vi "practice-01_thirteen segment display.vi"() -> ()   [LabVIEW 2015]
panel:
  out "Boolean 13":bool
  out "Boolean 12":bool
  out "Boolean 11":bool
  out "Boolean 3":bool
  out "Boolean 10":bool
  in  "stop 2":bool
  out "Boolean 6":bool
  out "Boolean 5":bool
  out "Boolean 7":bool
  out "Boolean 4":bool
  out "Boolean 8":bool
  out "Boolean 2":bool
  out "Boolean 9":bool
  in  "interlock":bool
  in  "emg2":bool
  in  "stop":bool
  in  "net":bool
  out "lamp":bool
  in  "emg1\nemg1":bool
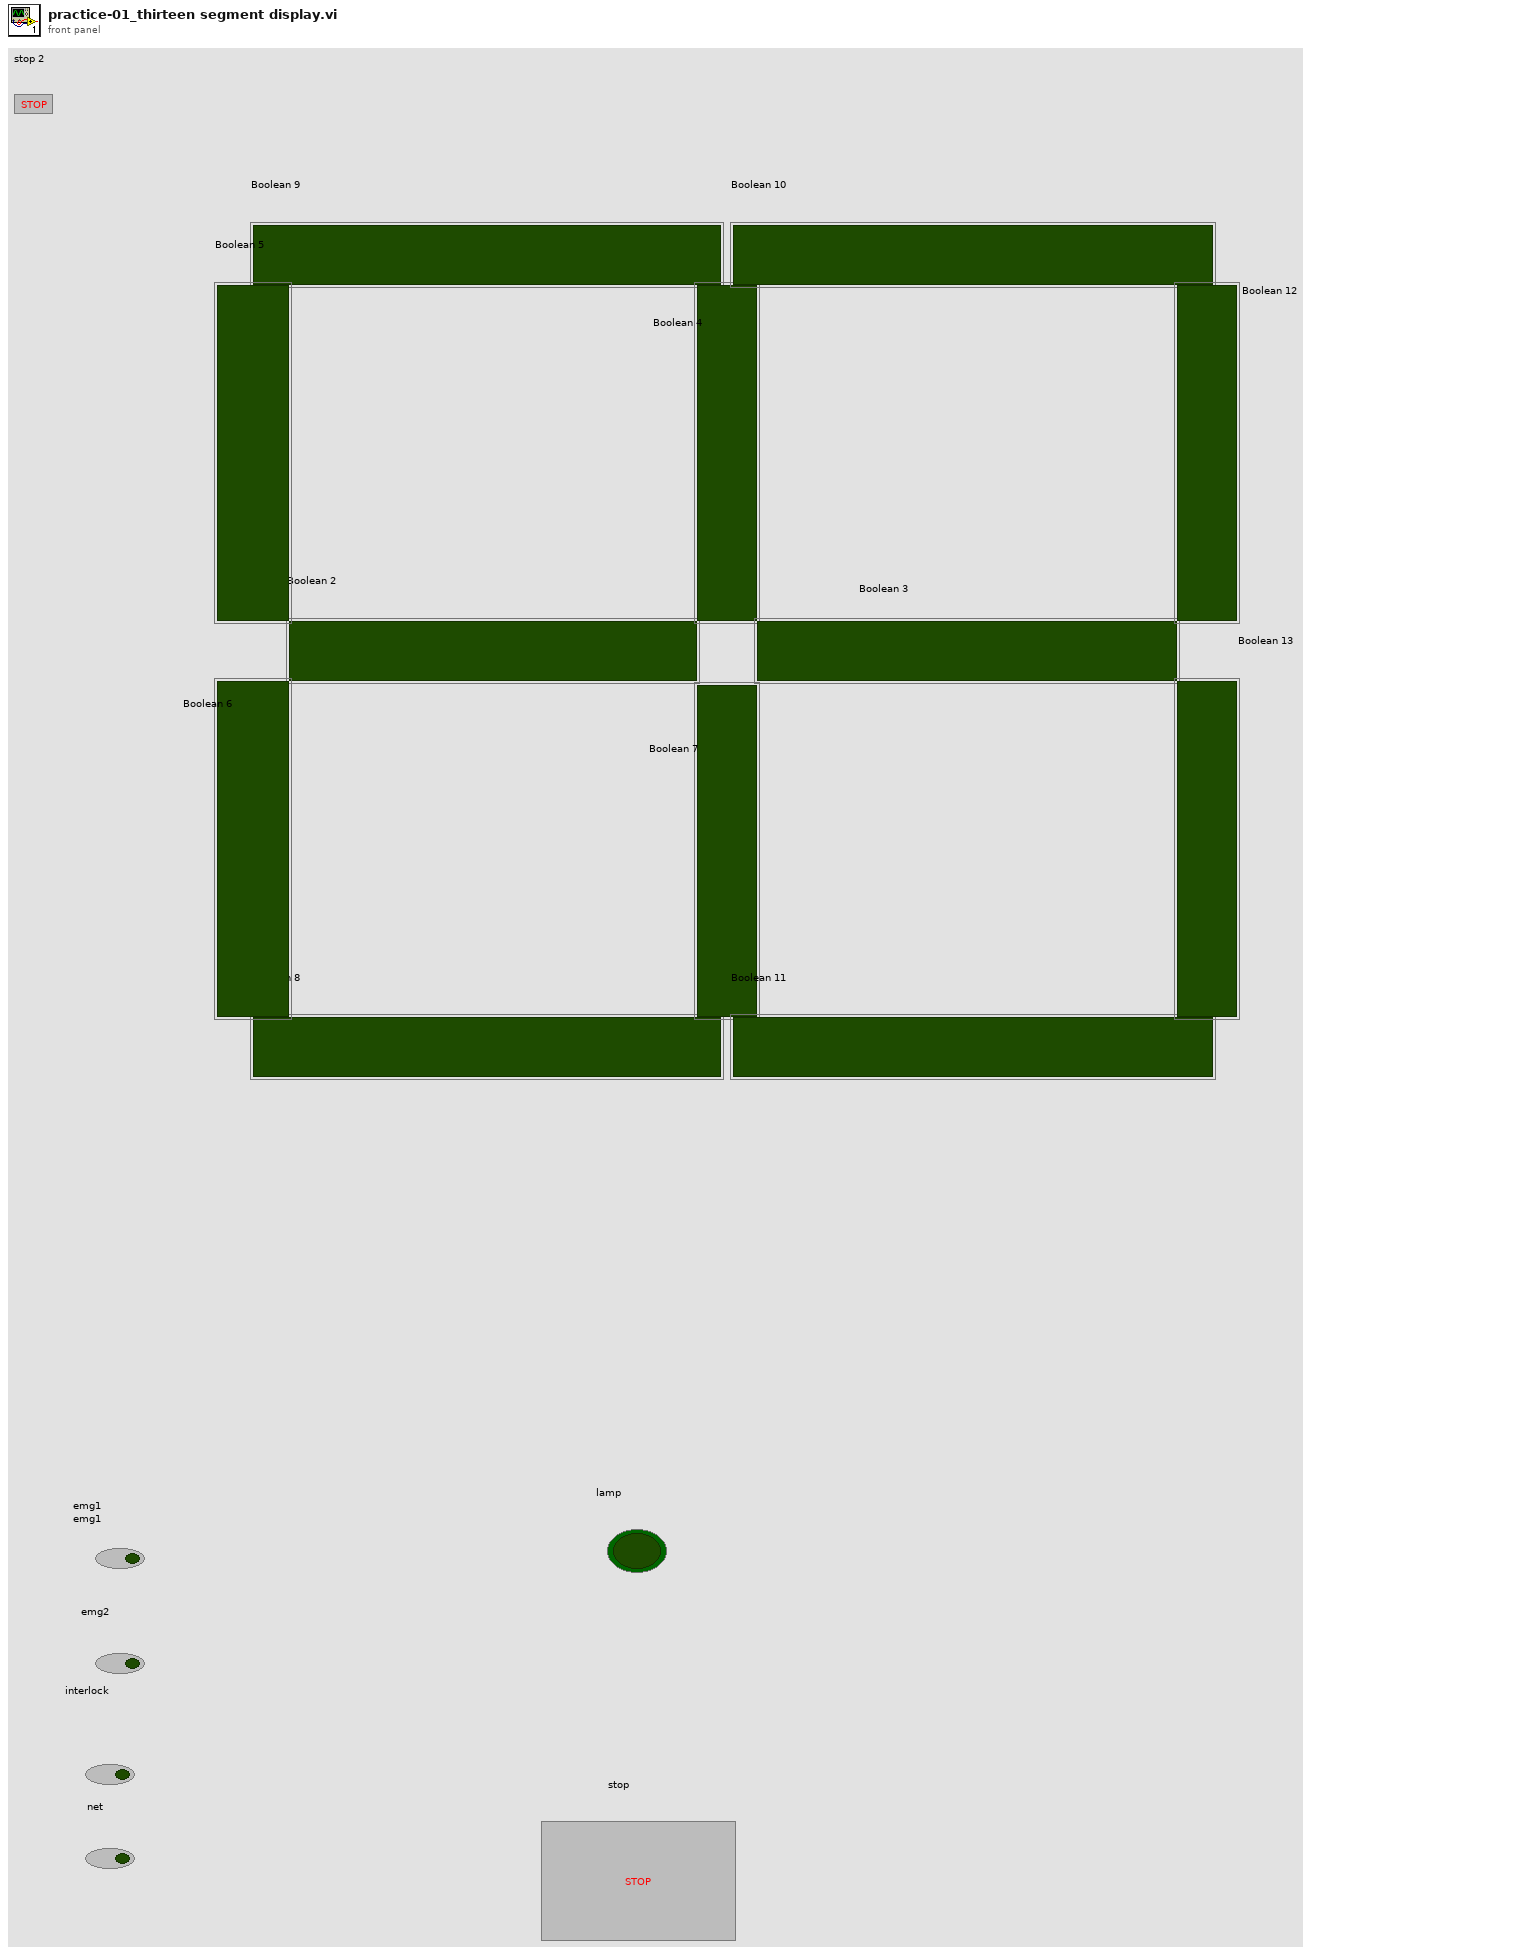
[diagram p1: front panel]
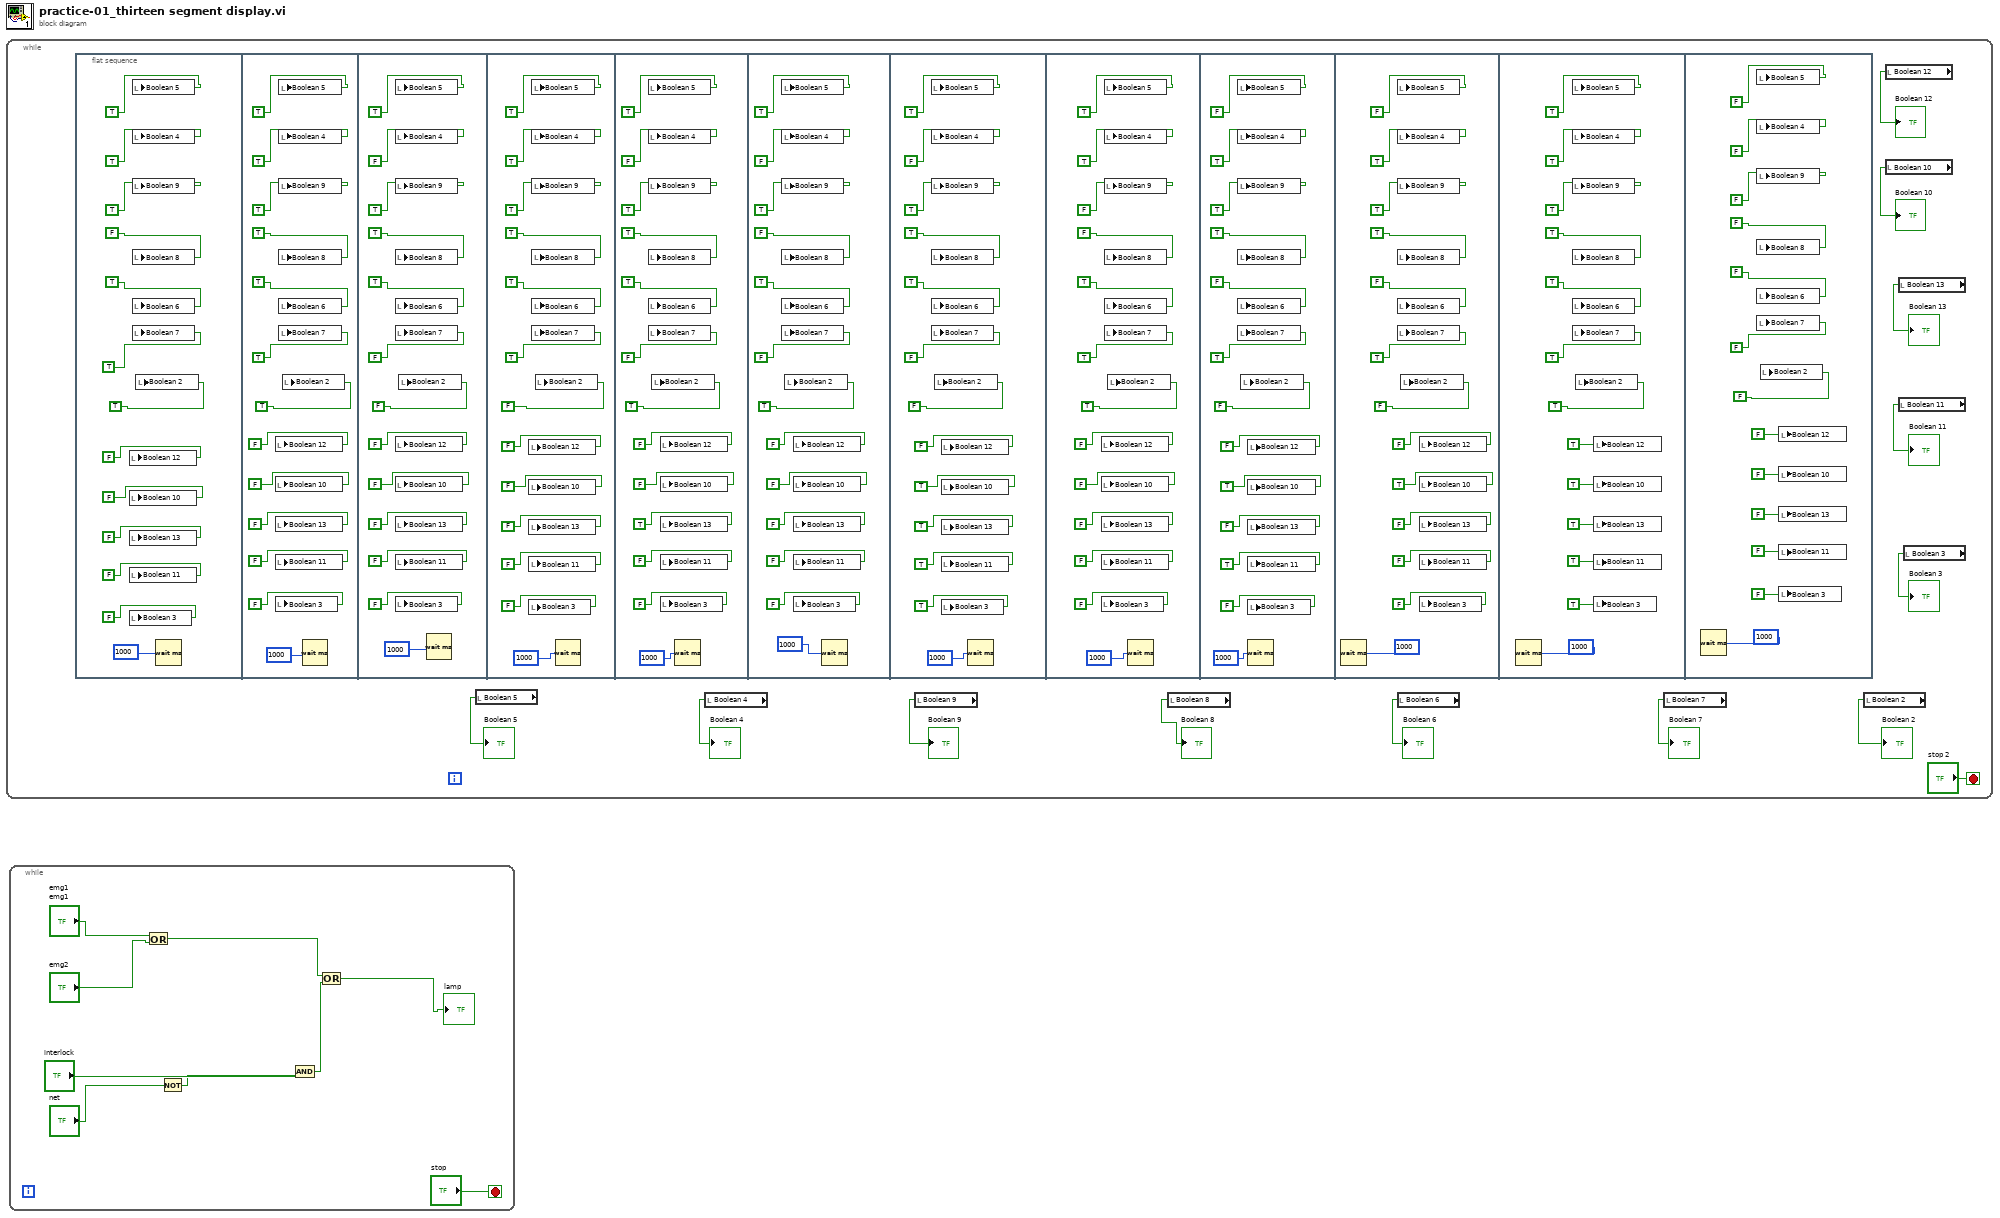
[diagram p0: block diagram]
diagram:
  n1 = while {
    stop <- "stop 2" stop-if-true
    n2 = flat-sequence {
      frame #0 {
        n3 = local write "Boolean 12"(FALSE ("Boolean 12")) -> ()
        n4 = local write "Boolean 10"(FALSE ("Boolean 10")) -> ()
        n5 = local write "Boolean 13"(FALSE ("Boolean 13")) -> ()
        n6 = local write "Boolean 11"(FALSE ("Boolean 11")) -> ()
        n7 = local write "Boolean 3"(FALSE ("Boolean 3")) -> ()
        n8 = local write "Boolean 5"(TRUE ("Boolean 5")) -> ()
        n9 = local write "Boolean 4"(TRUE ("Boolean 4")) -> ()
        n10 = local write "Boolean 9"(TRUE ("Boolean 9")) -> ()
        n11 = local write "Boolean 8"(FALSE ("Boolean 8")) -> ()
        n12 = local write "Boolean 6"(TRUE ("Boolean 5")) -> ()
        n13 = local write "Boolean 7"(TRUE ("Boolean 7")) -> ()
        n14 = local write "Boolean 2"(TRUE ("Boolean 2")) -> ()
        n15 = Wait (ms)(milliseconds to wait=u32 1000 ("millisecond timer value")) -> ()  [unwired: 1 out]
      }
      frame #1 {
        n16 = local write "Boolean 12"(FALSE ("Boolean 12")) -> ()
        n17 = local write "Boolean 10"(FALSE ("Boolean 10")) -> ()
        n18 = local write "Boolean 13"(FALSE ("Boolean 13")) -> ()
        n19 = local write "Boolean 11"(FALSE ("Boolean 11")) -> ()
        n20 = local write "Boolean 3"(FALSE ("Boolean 3")) -> ()
        n21 = local write "Boolean 5"(TRUE ("Boolean 5")) -> ()
        n22 = local write "Boolean 4"(TRUE ("Boolean 4")) -> ()
        n23 = local write "Boolean 9"(TRUE ("Boolean 9")) -> ()
        n24 = local write "Boolean 8"(TRUE ("Boolean 8")) -> ()
        n25 = local write "Boolean 6"(TRUE ("Boolean 5")) -> ()
        n26 = local write "Boolean 7"(TRUE ("Boolean 7")) -> ()
        n27 = local write "Boolean 2"(TRUE ("Boolean 2")) -> ()
        n28 = Wait (ms)(milliseconds to wait=u32 1000 ("millisecond timer value")) -> ()  [unwired: 1 out]
      }
      frame #2 {
        n29 = local write "Boolean 5"(TRUE ("Boolean 5")) -> ()
        n30 = local write "Boolean 4"(FALSE ("Boolean 4")) -> ()
        n31 = local write "Boolean 9"(TRUE ("Boolean 9")) -> ()
        n32 = local write "Boolean 8"(TRUE ("Boolean 8")) -> ()
        n33 = local write "Boolean 6"(TRUE ("Boolean 5")) -> ()
        n34 = local write "Boolean 7"(FALSE ("Boolean 7")) -> ()
        n35 = local write "Boolean 12"(FALSE ("Boolean 12")) -> ()
        n36 = local write "Boolean 10"(FALSE ("Boolean 10")) -> ()
        n37 = local write "Boolean 13"(FALSE ("Boolean 13")) -> ()
        n38 = local write "Boolean 11"(FALSE ("Boolean 11")) -> ()
        n39 = local write "Boolean 3"(FALSE ("Boolean 3")) -> ()
        n40 = local write "Boolean 2"(FALSE ("Boolean 2")) -> ()
        n41 = Wait (ms)(milliseconds to wait=u32 1000 ("millisecond timer value")) -> ()  [unwired: 1 out]
      }
      frame #3 {
        n42 = local write "Boolean 12"(FALSE ("Boolean 12")) -> ()
        n43 = local write "Boolean 10"(FALSE ("Boolean 10")) -> ()
        n44 = local write "Boolean 13"(FALSE ("Boolean 13")) -> ()
        n45 = local write "Boolean 11"(FALSE ("Boolean 11")) -> ()
        n46 = local write "Boolean 3"(FALSE ("Boolean 3")) -> ()
        n47 = local write "Boolean 5"(TRUE ("Boolean 5")) -> ()
        n48 = local write "Boolean 4"(TRUE ("Boolean 4")) -> ()
        n49 = local write "Boolean 9"(TRUE ("Boolean 9")) -> ()
        n50 = local write "Boolean 8"(TRUE ("Boolean 8")) -> ()
        n51 = local write "Boolean 6"(TRUE ("Boolean 5")) -> ()
        n52 = local write "Boolean 7"(TRUE ("Boolean 7")) -> ()
        n53 = local write "Boolean 2"(FALSE ("Boolean 2")) -> ()
        n54 = Wait (ms)(milliseconds to wait=u32 1000 ("millisecond timer value")) -> ()  [unwired: 1 out]
      }
      frame #4 {
        n55 = local write "Boolean 5"(TRUE ("Boolean 5")) -> ()
        n56 = local write "Boolean 4"(FALSE ("Boolean 4")) -> ()
        n57 = local write "Boolean 9"(TRUE ("Boolean 9")) -> ()
        n58 = local write "Boolean 8"(TRUE ("Boolean 8")) -> ()
        n59 = local write "Boolean 6"(TRUE ("Boolean 5")) -> ()
        n60 = local write "Boolean 7"(FALSE ("Boolean 7")) -> ()
        n61 = local write "Boolean 2"(TRUE ("Boolean 2")) -> ()
        n62 = local write "Boolean 12"(FALSE ("Boolean 12")) -> ()
        n63 = local write "Boolean 10"(FALSE ("Boolean 10")) -> ()
        n64 = local write "Boolean 13"(TRUE ("Boolean 13")) -> ()
        n65 = local write "Boolean 11"(FALSE ("Boolean 11")) -> ()
        n66 = local write "Boolean 3"(FALSE ("Boolean 3")) -> ()
        n67 = Wait (ms)(milliseconds to wait=u32 1000 ("millisecond timer value")) -> ()  [unwired: 1 out]
      }
      frame #5 {
        n68 = local write "Boolean 5"(TRUE ("Boolean 5")) -> ()
        n69 = local write "Boolean 4"(FALSE ("Boolean 4")) -> ()
        n70 = local write "Boolean 9"(TRUE ("Boolean 9")) -> ()
        n71 = local write "Boolean 8"(FALSE ("Boolean 8")) -> ()
        n72 = local write "Boolean 6"(TRUE ("Boolean 5")) -> ()
        n73 = local write "Boolean 7"(FALSE ("Boolean 7")) -> ()
        n74 = local write "Boolean 2"(TRUE ("Boolean 2")) -> ()
        n75 = local write "Boolean 12"(FALSE ("Boolean 12")) -> ()
        n76 = local write "Boolean 10"(FALSE ("Boolean 10")) -> ()
        n77 = local write "Boolean 13"(FALSE ("Boolean 13")) -> ()
        n78 = local write "Boolean 11"(FALSE ("Boolean 11")) -> ()
        n79 = local write "Boolean 3"(FALSE ("Boolean 3")) -> ()
        n80 = Wait (ms)(milliseconds to wait=u32 1000 ("millisecond timer value")) -> ()  [unwired: 1 out]
      }
      frame #6 {
        n81 = local write "Boolean 5"(TRUE ("Boolean 5")) -> ()
        n82 = local write "Boolean 4"(FALSE ("Boolean 4")) -> ()
        n83 = local write "Boolean 9"(TRUE ("Boolean 9")) -> ()
        n84 = local write "Boolean 8"(TRUE ("Boolean 8")) -> ()
        n85 = local write "Boolean 6"(TRUE ("Boolean 5")) -> ()
        n86 = local write "Boolean 7"(FALSE ("Boolean 7")) -> ()
        n87 = local write "Boolean 2"(FALSE ("Boolean 2")) -> ()
        n88 = local write "Boolean 12"(FALSE ("Boolean 12")) -> ()
        n89 = local write "Boolean 10"(TRUE ("Boolean 10")) -> ()
        n90 = local write "Boolean 13"(TRUE ("Boolean 13")) -> ()
        n91 = local write "Boolean 11"(TRUE ("Boolean 11")) -> ()
        n92 = local write "Boolean 3"(TRUE ("Boolean 3")) -> ()
        n93 = Wait (ms)(milliseconds to wait=u32 1000 ("millisecond timer value")) -> ()  [unwired: 1 out]
      }
      frame #7 {
        n94 = local write "Boolean 12"(FALSE ("Boolean 12")) -> ()
        n95 = local write "Boolean 10"(FALSE ("Boolean 10")) -> ()
        n96 = local write "Boolean 13"(FALSE ("Boolean 13")) -> ()
        n97 = local write "Boolean 11"(FALSE ("Boolean 11")) -> ()
        n98 = local write "Boolean 3"(FALSE ("Boolean 3")) -> ()
        n99 = local write "Boolean 5"(TRUE ("Boolean 5")) -> ()
        n100 = local write "Boolean 4"(TRUE ("Boolean 4")) -> ()
        n101 = local write "Boolean 9"(FALSE ("Boolean 9")) -> ()
        n102 = local write "Boolean 8"(FALSE ("Boolean 8")) -> ()
        n103 = local write "Boolean 6"(TRUE ("Boolean 5")) -> ()
        n104 = local write "Boolean 7"(TRUE ("Boolean 7")) -> ()
        n105 = local write "Boolean 2"(TRUE ("Boolean 2")) -> ()
        n106 = Wait (ms)(milliseconds to wait=u32 1000 ("millisecond timer value")) -> ()  [unwired: 1 out]
      }
      frame #8 {
        n107 = local write "Boolean 5"(FALSE ("Boolean 5")) -> ()
        n108 = local write "Boolean 4"(TRUE ("Boolean 4")) -> ()
        n109 = local write "Boolean 9"(TRUE ("Boolean 9")) -> ()
        n110 = local write "Boolean 8"(TRUE ("Boolean 8")) -> ()
        n111 = local write "Boolean 6"(FALSE ("Boolean 5")) -> ()
        n112 = local write "Boolean 7"(TRUE ("Boolean 7")) -> ()
        n113 = local write "Boolean 2"(FALSE ("Boolean 2")) -> ()
        n114 = local write "Boolean 12"(FALSE ("Boolean 12")) -> ()
        n115 = local write "Boolean 10"(TRUE ("Boolean 10")) -> ()
        n116 = local write "Boolean 13"(FALSE ("Boolean 13")) -> ()
        n117 = local write "Boolean 11"(TRUE ("Boolean 11")) -> ()
        n118 = local write "Boolean 3"(FALSE ("Boolean 3")) -> ()
        n119 = Wait (ms)(milliseconds to wait=u32 1000 ("millisecond timer value")) -> ()  [unwired: 1 out]
      }
      frame #9 {
        n120 = Wait (ms)(milliseconds to wait=u32 1000 ("millisecond timer value")) -> ()  [unwired: 1 out]
        n121 = local write "Boolean 5"(FALSE ("Boolean 5")) -> ()
        n122 = local write "Boolean 4"(TRUE ("Boolean 4")) -> ()
        n123 = local write "Boolean 9"(TRUE ("Boolean 9")) -> ()
        n124 = local write "Boolean 8"(TRUE ("Boolean 8")) -> ()
        n125 = local write "Boolean 6"(FALSE ("Boolean 5")) -> ()
        n126 = local write "Boolean 7"(TRUE ("Boolean 7")) -> ()
        n127 = local write "Boolean 2"(FALSE ("Boolean 2")) -> ()
        n128 = local write "Boolean 12"(FALSE ("Boolean 12")) -> ()
        n129 = local write "Boolean 10"(TRUE ("Boolean 10")) -> ()
        n130 = local write "Boolean 13"(FALSE ("Boolean 13")) -> ()
        n131 = local write "Boolean 11"(FALSE ("Boolean 11")) -> ()
        n132 = local write "Boolean 3"(FALSE ("Boolean 3")) -> ()
      }
      frame #10 {
        n133 = Wait (ms)(milliseconds to wait=u32 1000 ("millisecond timer value")) -> ()  [unwired: 1 out]
        n134 = local write "Boolean 5"(TRUE ("Boolean 5")) -> ()
        n135 = local write "Boolean 4"(TRUE ("Boolean 4")) -> ()
        n136 = local write "Boolean 9"(TRUE ("Boolean 9")) -> ()
        n137 = local write "Boolean 8"(TRUE ("Boolean 8")) -> ()
        n138 = local write "Boolean 6"(TRUE ("Boolean 5")) -> ()
        n139 = local write "Boolean 7"(TRUE ("Boolean 7")) -> ()
        n140 = local write "Boolean 2"(TRUE ("Boolean 2")) -> ()
        n141 = local write "Boolean 12"(TRUE ("Boolean 12")) -> ()
        n142 = local write "Boolean 10"(TRUE ("Boolean 10")) -> ()
        n143 = local write "Boolean 13"(TRUE ("Boolean 13")) -> ()
        n144 = local write "Boolean 11"(TRUE ("Boolean 11")) -> ()
        n145 = local write "Boolean 3"(TRUE ("Boolean 3")) -> ()
      }
      frame #11 {
        n146 = Wait (ms)(milliseconds to wait=u32 1000 ("millisecond timer value")) -> ()  [unwired: 1 out]
        n147 = local write "Boolean 5"(FALSE ("Boolean 5")) -> ()
        n148 = local write "Boolean 4"(FALSE ("Boolean 4")) -> ()
        n149 = local write "Boolean 9"(FALSE ("Boolean 9")) -> ()
        n150 = local write "Boolean 8"(FALSE ("Boolean 8")) -> ()
        n151 = local write "Boolean 6"(FALSE ("Boolean 5")) -> ()
        n152 = local write "Boolean 7"(FALSE ("Boolean 7")) -> ()
        n153 = local write "Boolean 2"(FALSE ("Boolean 2")) -> ()
        n154 = local write "Boolean 12"(FALSE ("Boolean 12")) -> ()
        n155 = local write "Boolean 10"(FALSE ("Boolean 10")) -> ()
        n156 = local write "Boolean 13"(FALSE ("Boolean 13")) -> ()
        n157 = local write "Boolean 11"(FALSE ("Boolean 11")) -> ()
        n158 = local write "Boolean 3"(FALSE ("Boolean 3")) -> ()
      }
    }
    n159 = local read "Boolean 5"() -> (→"Boolean 5":bool)
    n160 = local read "Boolean 4"() -> (→"Boolean 4":bool)
    n161 = local read "Boolean 9"() -> (→"Boolean 9":bool)
    n162 = local read "Boolean 8"() -> (→"Boolean 8":bool)
    n163 = local read "Boolean 6"() -> (→"Boolean 6":bool)
    n164 = local read "Boolean 7"() -> (→"Boolean 7":bool)
    n165 = local read "Boolean 2"() -> (→"Boolean 2":bool)
    n166 = local read "Boolean 12"() -> (→"Boolean 12":bool)
    n167 = local read "Boolean 10"() -> (→"Boolean 10":bool)
    n168 = local read "Boolean 13"() -> (→"Boolean 13":bool)
    n169 = local read "Boolean 11"() -> (→"Boolean 11":bool)
    n170 = local read "Boolean 3"() -> (→"Boolean 3":bool)
  }
  n171 = while {
    stop <- "stop" stop-if-true
    n172 = Or(x="emg1\nemg1", y="emg2") -> (x .or. y?=w176:bool)
    n173 = Not(x="net") -> (.not. x?=w172:bool)
    n174 = And(x="interlock", y=w172) -> (x .and. y?=w171:bool)
    n175 = Or(x=w176, y=w171) -> (x .or. y?=→"lamp":bool)
  }
